vi "Write Chnl.vi"(8 "error in (no error)":errorcluster, 10 "BME_DG_Chnl.lvclass":refnum<class "BME_DG_Chnl.lvclass">, 11 "BME_DG_System in":refnum<class "BME_DG_System.lvclass">) -> (0 "error out":errorcluster, 3 "BME_DG_System out":refnum<class "BME_DG_System.lvclass">)   [LabVIEW 2009, in "POLARIS BME DG.lvlib" / "BME_DG_System.lvclass"]
uses:
  BME_DG_System.lvclass
  BME_DG_Chnl/BME_DG_Chnl.lvclass
  BME_DG_Base/BME_DG_Base.lvclass
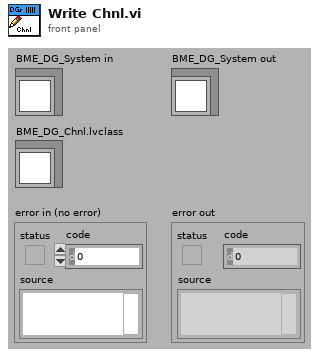
[diagram p1: front panel]
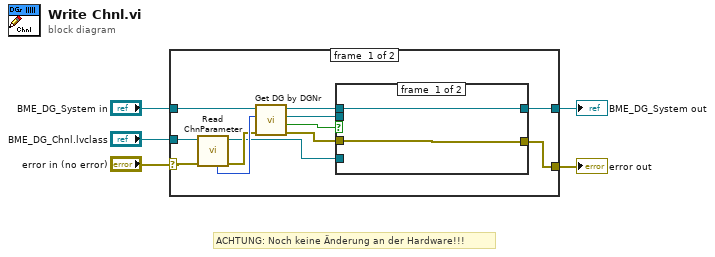
[diagram p0: block diagram]
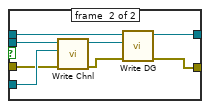
[diagram p2: hidden frame]
diagram:
  # "ACHTUNG: Noch keine Änderung an der Hardware!!!"
  n1 = case shown="No Error" "error in (no error)" {
    selector: "error in (no error)" -> [w13 w29]
    tunnel: [w6 w29] -> w4
    tunnel: [w8 w28] -> w2
    tunnel: "BME_DG_System in" -> [w16 w28]
    tunnel: "BME_DG_Chnl.lvclass" -> [w17 _]
    frame #0 {
      n2 = call-dynamic "Read ChnParameter.vi"("error in (no error)"=w13, "BME_DG_Chnl in"=w17) -> ("error out"=w12:errorcluster, "BME_DG_Chnl out"=w10:refnum<class "BME_DG_Chnl.lvclass">, "DG Nr"=w14:i32)  [unwired: 4 in, 3 out]
      n3 = call "Get DG by DGNr.vi"("error in (no error)"=w12, "DG Nr."=w14, "BME_DG_System in"=w16) -> ("error out"=w7:errorcluster, "found?"=w15:bool, "BME_DG_Base.lvclass"=w11:refnum<class "BME_DG_Base.lvclass">, "BME_DG_System out"=w9:refnum<class "BME_DG_System.lvclass">)  [unwired: 5 in]
      n4 = case shown="True" w15 {
        tunnel: w11 -> [_ w27]
        tunnel: w10 -> [_ w26]
        tunnel: w9 -> [w19 w23]
        tunnel: [w19 w24] -> w8
        tunnel: w7 -> [w18 w25]
        tunnel: [w18 w20] -> w6
        frame #0 {
        }
        frame #1 {
          n5 = call-dynamic "Write Chnl.vi"("error in (no error)"=w25, "BME_DG_Chnl"=w26, "BME_DG_Base in"=w27) -> ("error out"=w21:errorcluster, "BME_DG_Base out"=w22:refnum<class "BME_DG_Base.lvclass">)  [unwired: 7 in]
          n6 = call "Write DG.vi"("error in (no error)"=w21, "BME_DG_Base"=w22, "BME_DG_System in"=w23) -> ("error out"=w20:errorcluster, "BME_DG_System out"=w24:refnum<class "BME_DG_System.lvclass">)  [unwired: 7 in]
        }
      }
    }
    frame #1 {
    }
  }
  "error out" <- w4
  "BME_DG_System out" <- w2
